vi "CalculateAngles.vi"(8 "error in (no error)":errorcluster, 11 "reference in":refnum<class "Manipulator.lvclass">) -> (0 "error out":errorcluster, 3 "reference out":refnum<class "Manipulator.lvclass">)   [LabVIEW 2014, in "Manipulator.lvclass"]
uses:
  Manipulator.lvclass
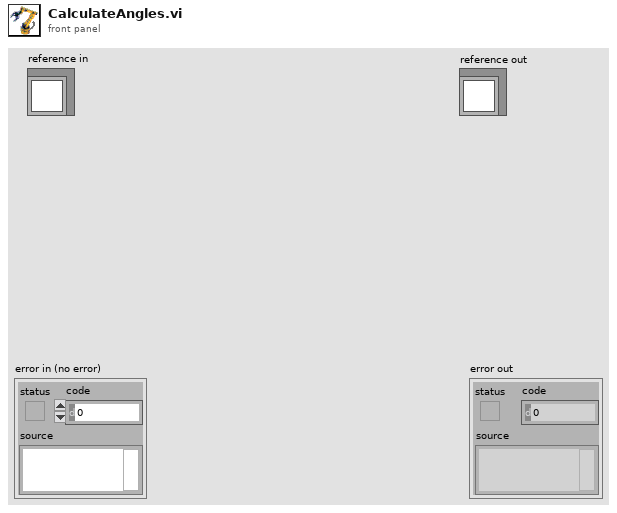
[diagram p1: front panel]
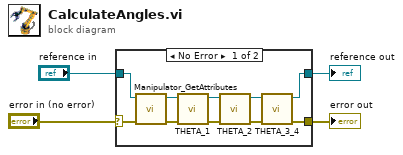
[diagram p0: block diagram]
diagram:
  n1 = case shown="No Error" "error in (no error)" {
    selector: "error in (no error)" -> [w13 w16]
    tunnel: [w5 w16] -> w3
    tunnel: [w6 w15] -> w1
    tunnel: "reference in" -> [w14 w15]
    frame No Error {
      n2 = call "Manipulator_GetAttributes.vi"("error in (no error)"=w13, "reference in"=w14) -> ("error out"=w11:errorcluster, "reference out"=w12:refnum<class "Manipulator.lvclass">)  [unwired: 6 in, 2 out]
      n3 = call "THETA_1.vi"("error in (no error)"=w11, "reference in"=w12) -> ("error out"=w9:errorcluster, "reference out"=w10:refnum<class "Manipulator.lvclass">)  [unwired: 7 in, 1 out]
      n4 = call "THETA_2.vi"("error in (no error)"=w9, "reference in"=w10) -> ("error out"=w8:errorcluster, "reference out"=w7:refnum<class "Manipulator.lvclass">)  [unwired: 8 in]
      n5 = call "THETA_3_4.vi"("error in (no error)"=w8, "reference in"=w7) -> ("error out"=w5:errorcluster, "reference out"=w6:refnum<class "Manipulator.lvclass">)  [unwired: 8 in]
    }
    frame Error {
    }
  }
  "error out" <- w3
  "reference out" <- w1
